vi "DecodeConsole.vi"(10 "Boolean Array":bool[](array[boolean]), 11 "Axis Array":dbl[](array[numeric])) -> (2 "Wrist":T2(ring), 3 "Elevator Level Select":T1(ring))   [LabVIEW 2018]
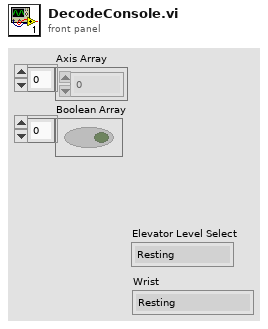
[diagram p1: front panel]
types:
  T1 = enum16{"Resting", "CargoShip Front", "CargoShip Back", "Cargo Mid", "Hatch Mid", "All High", "Cargo Intake"}
  T2 = enum16{"Resting", "Hatch Ground Intake", "Hatch Place Low/Mid/CargoShip", "Hatch Place High", "Cargo Ground Intake", "Cargo Place Low/Mid", "Cargo Place High", "CargoShip Place Front", "CargoShip Place Back"}
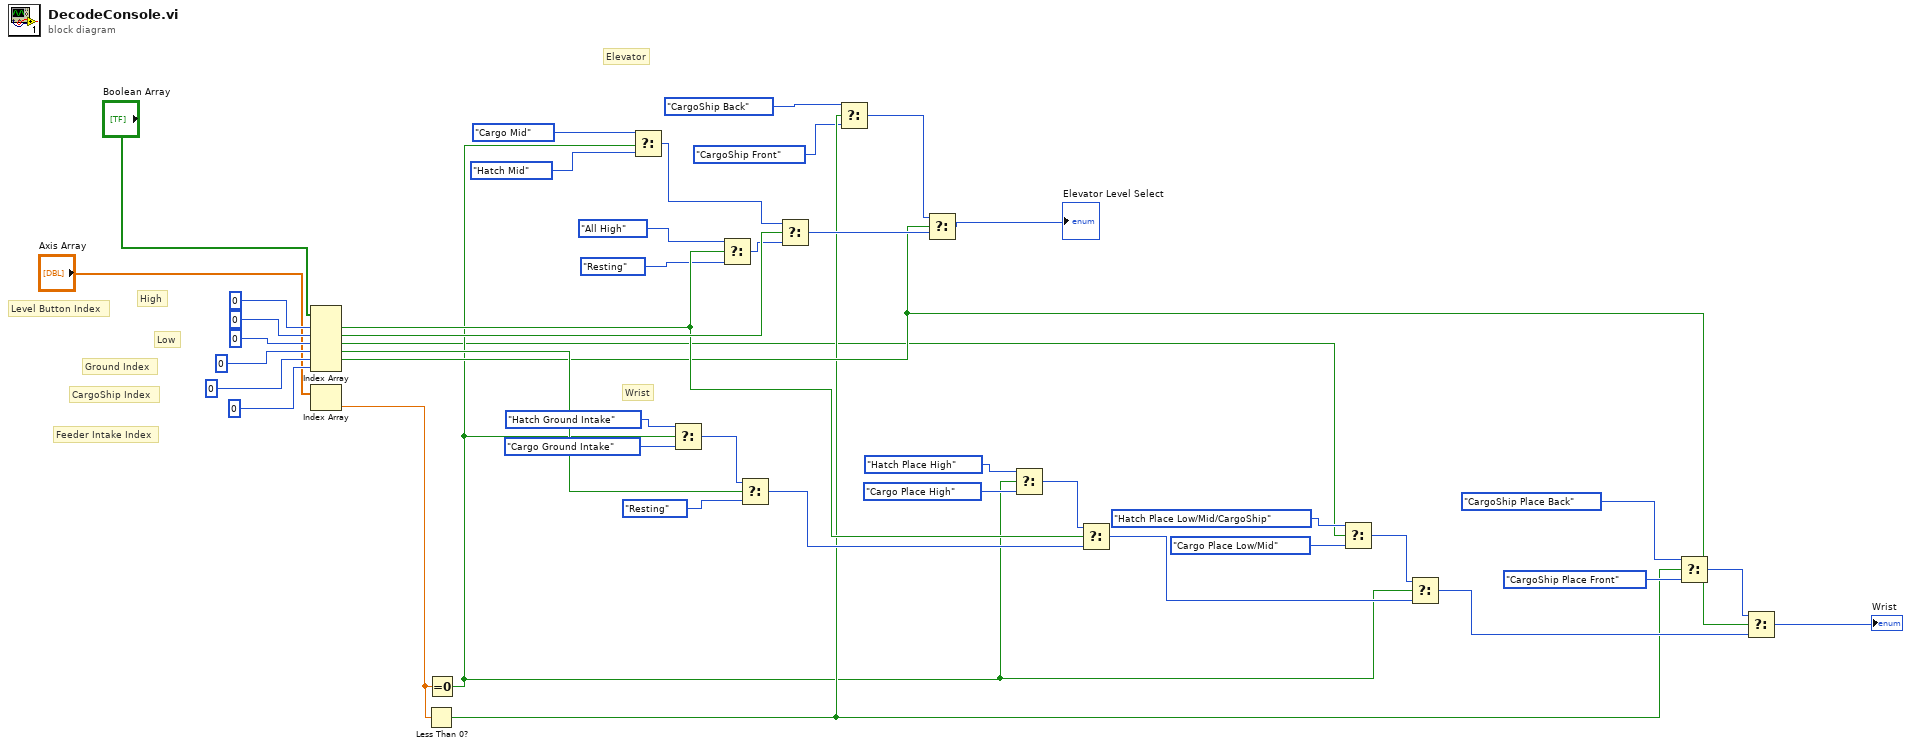
[diagram p0: block diagram]
diagram:
  # "Elevator"
  # "Wrist"
  # "CargoShip Index"
  # "Low"
  # "High"
  # "Feeder Intake Index"
  # "Ground Index"
  # "Level Button Index"
  n1 = Index Array(array="Boolean Array", index #1=0 ("index"), index #2=0 ("index"), index #3=0 ("index"), index #4=0 ("index"), index #5=0 ("index"), index #6=0 ("index")) -> (element #1=w23:bool, element #2=w38:bool, element #3=w9:bool, element #4=w32:bool, element #5=w13:bool)  [unwired: 1 out]
  n2 = Index Array(array="Axis Array") -> (element=w15:dbl)  [unwired: 1 in]
  n3 = Less Than 0?(x=w15) -> (x < 0?=w11:bool)
  n4 = Equal To 0?(x=w15) -> (x = 0?=w10:bool)
  n5 = Select(t=T1."Cargo Mid" ("Elevator Level Select"), s=w10, f=T1."Hatch Mid" ("Elevator Level Select")) -> (s? t:f=w35:T1)
  n6 = Select(t=T2."Hatch Ground Intake" ("Wrist"), s=w10, f=T2."Cargo Ground Intake" ("Wrist")) -> (s? t:f=w29:T2)
  n7 = Select(t=T1."All High" ("Elevator Level Select"), s=w23, f=T1."Resting" ("Elevator Level Select")) -> (s? t:f=w37:T1)
  n8 = Select(t=w29, s=w32, f=T2."Resting") -> (s? t:f=w24:T2)
  n9 = Select(t=w35, s=w38, f=w37) -> (s? t:f=w34:T1)
  n10 = Select(t=T1."CargoShip Back" ("Elevator Level Select"), s=w11, f=T1."CargoShip Front" ("Elevator Level Select")) -> (s? t:f=w33:T1)
  n11 = Select(t=w33, s=w13, f=w34) -> (s? t:f=→"Elevator Level Select":T1)
  n12 = Select(t=T2."Hatch Place High" ("Wrist"), s=w10, f=T2."Cargo Place High" ("Wrist")) -> (s? t:f=w25:T2)
  n13 = Select(t=w25, s=w23, f=w24) -> (s? t:f=w19:T2)
  n14 = Select(t=T2."Hatch Place Low/Mid/CargoShip" ("Wrist"), s=w9, f=T2."Cargo Place Low/Mid" ("Wrist")) -> (s? t:f=w20:T2)
  n15 = Select(t=w20, s=w10, f=w19) -> (s? t:f=w14:T2)
  n16 = Select(t=T2."CargoShip Place Back" ("Wrist"), s=w11, f=T2."CargoShip Place Front" ("Wrist")) -> (s? t:f=w16:T2)
  n17 = Select(t=w16, s=w13, f=w14) -> (s? t:f=→"Wrist":T2)
